vi "struct_ads_vol_dA_dW_WRho.vi"(8 "Error (Input)":errorcluster, 9 "Saturated liquid density of adsorpt rho_l in kg/m3 (Input)":dbl, 10 "Volumetric loading W in m3/kg (Input)":dbl, 11 "Reference working pair (Input)":i64) -> (0 "Error (Output)":errorcluster caption="Error(Output)", 3 "Der. of adsorption potential wrt. volumetric loading in kgJ/mol/m3 (Output)":dbl)   [LabVIEW 2017]
doc: "ads_vol_dA_dW_WRho:\n * -------------------\n *\n * Calculates derivative of equilibrium adsorption potential dA_dW in kgJ/mol/m³\n * depending on equilibrium volumetric loading W in m³/kg and saturated liquid\n * density of adsorpt rho_l in kg/m3.\n *\n * Parameters:\n * -----------\n * double W_m3kg:\n * Equilibrium volumetric loading W in m³/kg.\n * double rho_l_kgm3:\n * Saturated liquid density of adsorpt rho_l in kg/m3.\n * struct *WorkingPair:\n * Pointer of WorkingPair-struct.\n *\n * Returns:\n * --------\n * double:\n * Derivative of adsorption potential wrt. volumetric loading in\n * kgJ/mol/m³.\n *\n * Remarks:\n * --------\n * This function is only valid for isotherm models based on the volumetric\n * approach.\n * Saturated liquid density of adsorpt is required to calculate volumetric\n * loading from characteristic curve in m3/kg when coefficients would directly\n * return loading w in kg/kg.\n *\n * History:\n * --------\n * 07/07/2021, by Jannik Driesel (supervised by Mirko Engelpracht):\n * First implementation."
uses:
  data/win32bit/libsorpPropLib.dll
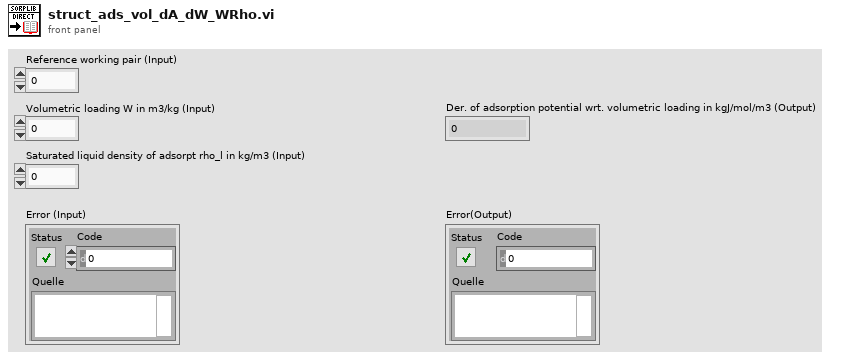
[diagram p1: front panel]
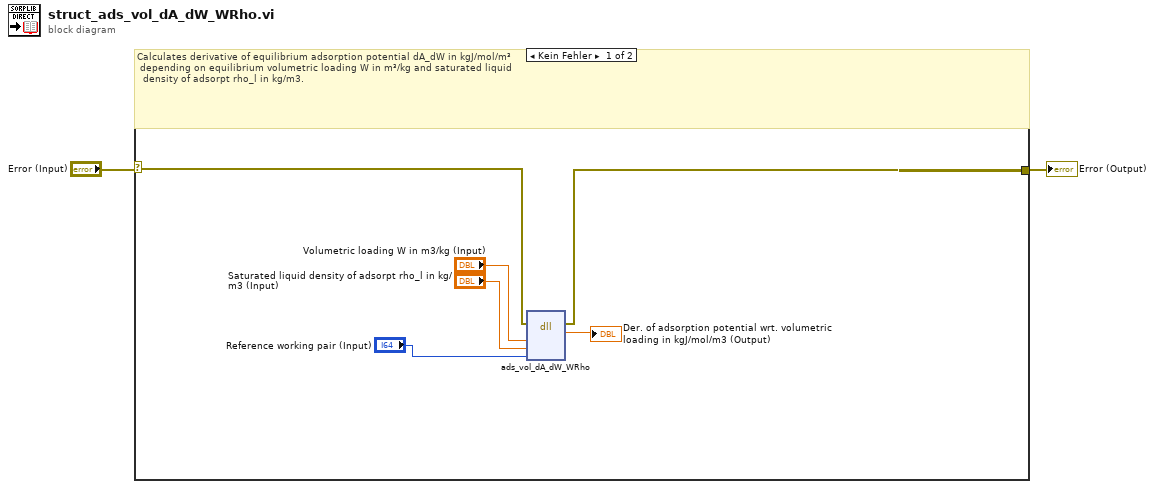
[diagram p0: block diagram]
diagram:
  n1 = case shown="Kein Fehler" "Error (Input)" {
    selector: "Error (Input)" -> [w7 w9]
    tunnel: [w6 w9] -> w1
    frame No Error {
      # "Calculates derivative of equilibrium adsorption potential dA_dW in kgJ/mol/m³\n depending on equilibrium volumetric loading W in m³/kg and saturated liquid\n  density of adsorpt rho_l in kg/m3."
      n2 = dll-call lib="D:/Driesel/SorpLibLocal/LabVIEW_wrapper/data/win32bit/libsorpPropLib.dll" fn="ads_vol_dA_dW_WRho"(error in=w7, "W_m3kg"="Volumetric loading W in m3/kg (Input)", "rho_l_kgm3"="Saturated liquid density of adsorpt rho_l in kg/m3 (Input)", "workingPair"="Reference working pair (Input)") -> (error out=w6:errorcluster, "dA_dW_kgJmolm3"=→"Der. of adsorption potential wrt. volumetric loading in kgJ/mol/m3 (Output)":dbl)  [unwired: 5 in, 1 out]
    }
    frame Error {
      # "Error - No calculations"
    }
  }
  "Error (Output)" <- w1
